vi "dependencies.vi"(8 "error in (no error)":errorcluster, 11 "lv-builder-default in":refnum<class "lv-builder-default.lvclass">) -> (0 "error out":errorcluster, 3 "lv-builder-default out":refnum<class "lv-builder-default.lvclass">)   [LabVIEW 2015, in "lv-builder-default.lvclass"]
uses:
  lv-builder-default.lvclass
  lv-builder-default.lvlib
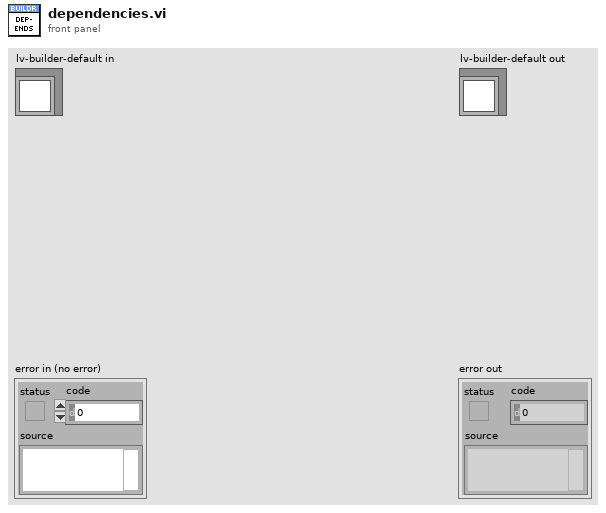
[diagram p1: front panel]
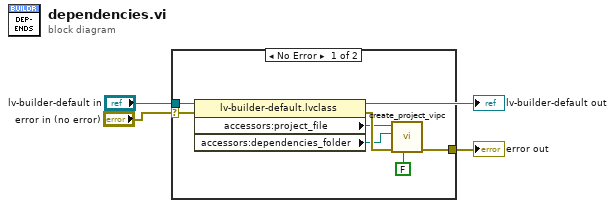
[diagram p0: block diagram]
diagram:
  n1 = case shown="No Error" "error in (no error)" {
    selector: "error in (no error)" -> [w4 w11]
    tunnel: "lv-builder-default in" -> [w8 _]
    tunnel: [w5 w11] -> w3
    frame No Error {
      n2 = property class="lv-builder-default.lvclass"(reference=w8, error in=w4) -> (error out=w10:errorcluster, "accessors:project_file"=w7:path, "accessors:dependencies_folder"=w6:path)  [unwired: 1 out]
      n3 = call "create_project_vipc.vi"("quet"=FALSE ("quiet? (T)"), "error in (no error)"=w10, "dependencies_folder"=w6, "project_file"=w7) -> ("error out"=w5:errorcluster)  [unwired: 7 in]
    }
    frame Error {
    }
  }
  "error out" <- w3
  "lv-builder-default out" <- "lv-builder-default in"
